vi "autocorrelator-test.vi"() -> ()   [LabVIEW 2011]
uses:
  <vilib>/Waveform/WDTOps.llb/WDT Get XY Value DBL.vi
  <vilib>/Utility/file.llb/Write To Spreadsheet File (DBL).vi
panel:
  in  "file path (dialog if empty)":path
  in  "stop":bool
  out "XY Graph 2":cluster{sgl[], dbl[]}(graph)={[7.5546875, 7.5564947, 7.5579815, 7.559002, 7.5601096, 7.5602555, 7.5602264, 7.559235, 7.5582147, 7.5566406, 7.5546875, 7.552297, 7.5473995, 7.5458837, 7.542823, 7.5388584, 7.534661, 7.530113, 7.524866, 7.519502, 7.5128264, 7.5075793, 7.500583, 7.4940534, 7.4866195, 7.4764752, 7.4705863, 7.4628615, 7.454874, 7.446333, 7.4387536, 7.425752, 7.422225, 7.4146457, 7.4067745, 7.3987875, 7.390654, 7.3826666, 7.3743877, 7.366255, 7.3585587, 7.350513, 7.34238, 7.334655, 7.324598, 7.3181844, 7.310605, 7.302647, 7.294572, 7.286468, 7.274108, 7.270406, 7.2626514, 7.253411, 7.246385, 7.2385726, 7.229361, 7.2227144, 7.2142606, 7.206565, 7.1987233, 7.18922, 7.1825733, 7.1745567, 7.1656075, 7.158582, 7.150449, 7.142607, 7.1346197, 7.1264286, 7.1174207, 7.1103954, 7.102554, 7.0946245, 7.0863748, 7.078533, 7.070633, 7.061917, 7.0544543, 7.046321, 7.038567, 7.0305214, 7.0214844, 7.014138, 7.0066757, 6.997668, 6.9904966, 6.982684, 6.973414, 6.9660974, 6.958576, 6.9507637, 6.942514, 6.9347014, 6.926656, 6.918464, 6.910681, 6.9021688, 6.8945603, 6.8868356, 6.878615, 6.8707733, 6.861299, 6.85474, 6.8466945, 6.838736, 6.8305736, 6.822761, 6.8135204, 6.8067575, 6.798537, 6.7908115, 6.7826786, 6.774662, 6.7665286, 6.7582207, 6.7506413, 6.7427416, 6.7348123, 6.7264752, 6.7184587, 6.7094216, 6.7025127, 6.694584, 6.685372, 6.678667, 6.6677938, 6.661585, 6.65488, 6.6468635, 6.638759, 6.630597, 6.6173334, 6.614331, 6.605848, 6.598414, 6.590631, 6.58276, 6.574773, 6.5666103, 6.557282, 6.5507812, 6.5426483, 6.534923, 6.5267024, 6.5162373, 6.510086, 6.5027695, 6.494549, 6.485337, 6.478603, 6.4657183, 6.4614916, 6.454466, 6.4466243, 6.438841, 6.430679, 6.4228663, 6.4146166, 6.4059877, 6.398904, 6.3908, 6.3826957, 6.374621, 6.364797, 6.357568, 6.350746, 6.341593, 6.334859, 6.326726, 6.314191, 6.310372, 6.3027344, 6.2948346, 6.286789, 6.2786264, 6.2707267, 6.2627683, 6.2544894, 6.246881, 6.2388935, 6.230673, 6.2226853, 6.213328, 6.206711, 6.1988688, 6.189628, 6.1829524, 6.174761, 6.166832, 6.1586695, 6.150799, 6.142345, 6.1345906, 6.126807, 6.118645, 6.110891, 6.1032825, 6.095616, 6.0896106, 6.083401, 6.0774837, 6.071245, 6.0667562], array[204 elements]}
  out "XY Graph":cluster{sgl[], dbl[]}(graph)={[6.06078, 6.0535216, 6.0500236, 6.045476, 6.043464, 6.041482, 6.0394416, 6.0375757, 6.036381, 6.0350103, 6.034865, 6.034748, 6.034486, 6.0351562, 6.036089, 6.0373716, 6.0391793, 6.041278, 6.043523, 6.046642, 6.0500236, 6.053842, 6.059585, 6.062704, 6.0670185, 6.073169, 6.077921, 6.0840716, 6.090223, 6.097569, 6.1042733, 6.11299, 6.119549, 6.127711, 6.135611, 6.144036, 6.1519938, 6.159573, 6.1677647, 6.175694, 6.1847305, 6.194555, 6.1999183, 6.207964, 6.2158055, 6.223764, 6.2316346, 6.2450733, 6.247843, 6.2556844, 6.264255, 6.2716885, 6.279851, 6.2877216, 6.2958837, 6.304046, 6.3117423, 6.3197293, 6.327775, 6.337162, 6.3461404, 6.3521748, 6.361182, 6.367887, 6.3758745, 6.3849697, 6.3967175, 6.400857, 6.4088445, 6.4162197, 6.423974, 6.432865, 6.4400363, 6.4480233, 6.4571185, 6.463882, 6.4719567, 6.4796233, 6.487844, 6.4978137, 6.5056553, 6.511806, 6.5197935, 6.52781, 6.5358267, 6.548274, 6.5519767, 6.5598764, 6.568884, 6.5757055, 6.583897, 6.5943913, 6.600455, 6.608034, 6.6169834, 6.6240964, 6.631938, 6.6409163, 6.647971, 6.6561627, 6.6638002, 6.671758, 6.6798625, 6.689045, 6.699802, 6.7040286, 6.711695, 6.719887, 6.727816, 6.736707, 6.743645, 6.7518363, 6.7603197, 6.767607, 6.775682, 6.7838736, 6.792007, 6.7997026, 6.807836, 6.815736, 6.8237233, 6.8325267, 6.8398438, 6.8513584, 6.857043, 6.8639517, 6.871706, 6.8812094, 6.887739, 6.89561, 6.9042096, 6.911614, 6.920709, 6.9277053, 6.935809, 6.9447002, 6.952542, 6.960267, 6.9682837, 6.975571, 6.9837337, 6.991721, 7.0029445, 7.0082498, 7.015771, 7.0250115, 7.0316, 7.039704, 7.053492, 7.0564365, 7.0637245, 7.0716243, 7.079874, 7.0878325, 7.0962863, 7.10404, 7.1119986, 7.1208024, 7.1276526, 7.13564, 7.1435986, 7.154559, 7.159952, 7.1677938, 7.1756644, 7.1837397, 7.1916103, 7.205049, 7.2078767, 7.2155433, 7.223589, 7.2315764, 7.2408175, 7.2474346, 7.255626, 7.265071, 7.2714844, 7.279734, 7.2875757, 7.2956505, 7.3059993, 7.3134913, 7.319671, 7.3276877, 7.3355002, 7.3436627, 7.3565183, 7.360745, 7.367945, 7.3757286, 7.383804, 7.391587, 7.399691, 7.4075327, 7.4162197, 7.423741, 7.4315534, 7.4397154, 7.447674, 7.4574685, 7.463911, 7.4716067, 7.479419, 7.4873486, 7.4944906, 7.50516, 7.5080166, 7.5155377, 7.5203185, 7.5253906, 7.530113, 7.534923, 7.5392375, 7.543027, 7.5464377, 7.5495276, 7.552064], array[217 elements]}
  out "Waveform Graph 2":sgl[](graph)=[7.5546875, 7.5564947, 7.5579815, 7.559002, 7.5601096, 7.5602555, 7.5602264, 7.559235, 7.5582147, 7.5566406, 7.5546875, 7.552297, 7.5473995, 7.5458837, 7.542823, 7.5388584, 7.534661, 7.530113, 7.524866, 7.519502, 7.5128264, 7.5075793, 7.500583, 7.4940534, 7.4866195, 7.4764752, 7.4705863, 7.4628615, 7.454874, 7.446333, 7.4387536, 7.425752, 7.422225, 7.4146457, 7.4067745, 7.3987875, 7.390654, 7.3826666, 7.3743877, 7.366255, 7.3585587, 7.350513, 7.34238, 7.334655, 7.324598, 7.3181844, 7.310605, 7.302647, 7.294572, 7.286468, 7.274108, 7.270406, 7.2626514, 7.253411, 7.246385, 7.2385726, 7.229361, 7.2227144, 7.2142606, 7.206565, 7.1987233, 7.18922, 7.1825733, 7.1745567, 7.1656075, 7.158582, 7.150449, 7.142607, 7.1346197, 7.1264286, 7.1174207, 7.1103954, 7.102554, 7.0946245, 7.0863748, 7.078533, 7.070633, 7.061917, 7.0544543, 7.046321, 7.038567, 7.0305214, 7.0214844, 7.014138, 7.0066757, 6.997668, 6.9904966, 6.982684, 6.973414, 6.9660974, 6.958576, 6.9507637, 6.942514, 6.9347014, 6.926656, 6.918464, 6.910681, 6.9021688, 6.8945603, 6.8868356, 6.878615, 6.8707733, 6.861299, 6.85474, 6.8466945, 6.838736, 6.8305736, 6.822761, 6.8135204, 6.8067575, 6.798537, 6.7908115, 6.7826786, 6.774662, 6.7665286, 6.7582207, 6.7506413, 6.7427416, 6.7348123, 6.7264752, 6.7184587, 6.7094216, 6.7025127, 6.694584, 6.685372, 6.678667, 6.6677938, 6.661585, 6.65488, 6.6468635, 6.638759, 6.630597, 6.6173334, 6.614331, 6.605848, 6.598414, 6.590631, 6.58276, 6.574773, 6.5666103, 6.557282, 6.5507812, 6.5426483, 6.534923, 6.5267024, 6.5162373, 6.510086, 6.5027695, 6.494549, 6.485337, 6.478603, 6.4657183, 6.4614916, 6.454466, 6.4466243, 6.438841, 6.430679, 6.4228663, 6.4146166, 6.4059877, 6.398904, 6.3908, 6.3826957, 6.374621, 6.364797, 6.357568, 6.350746, 6.341593, 6.334859, 6.326726, 6.314191, 6.310372, 6.3027344, 6.2948346, 6.286789, 6.2786264, 6.2707267, 6.2627683, 6.2544894, 6.246881, 6.2388935, 6.230673, 6.2226853, 6.213328, 6.206711, 6.1988688, 6.189628, 6.1829524, 6.174761, 6.166832, 6.1586695, 6.150799, 6.142345, 6.1345906, 6.126807, 6.118645, 6.110891, 6.1032825, 6.095616, 6.0896106, 6.083401, 6.0774837, 6.071245, 6.0667562]
  out "Waveform Graph":sgl[](graph)=[6.06078, 6.0535216, 6.0500236, 6.045476, 6.043464, 6.041482, 6.0394416, 6.0375757, 6.036381, 6.0350103, 6.034865, 6.034748, 6.034486, 6.0351562, 6.036089, 6.0373716, 6.0391793, 6.041278, 6.043523, 6.046642, 6.0500236, 6.053842, 6.059585, 6.062704, 6.0670185, 6.073169, 6.077921, 6.0840716, 6.090223, 6.097569, 6.1042733, 6.11299, 6.119549, 6.127711, 6.135611, 6.144036, 6.1519938, 6.159573, 6.1677647, 6.175694, 6.1847305, 6.194555, 6.1999183, 6.207964, 6.2158055, 6.223764, 6.2316346, 6.2450733, 6.247843, 6.2556844, 6.264255, 6.2716885, 6.279851, 6.2877216, 6.2958837, 6.304046, 6.3117423, 6.3197293, 6.327775, 6.337162, 6.3461404, 6.3521748, 6.361182, 6.367887, 6.3758745, 6.3849697, 6.3967175, 6.400857, 6.4088445, 6.4162197, 6.423974, 6.432865, 6.4400363, 6.4480233, 6.4571185, 6.463882, 6.4719567, 6.4796233, 6.487844, 6.4978137, 6.5056553, 6.511806, 6.5197935, 6.52781, 6.5358267, 6.548274, 6.5519767, 6.5598764, 6.568884, 6.5757055, 6.583897, 6.5943913, 6.600455, 6.608034, 6.6169834, 6.6240964, 6.631938, 6.6409163, 6.647971, 6.6561627, 6.6638002, 6.671758, 6.6798625, 6.689045, 6.699802, 6.7040286, 6.711695, 6.719887, 6.727816, 6.736707, 6.743645, 6.7518363, 6.7603197, 6.767607, 6.775682, 6.7838736, 6.792007, 6.7997026, 6.807836, 6.815736, 6.8237233, 6.8325267, 6.8398438, 6.8513584, 6.857043, 6.8639517, 6.871706, 6.8812094, 6.887739, 6.89561, 6.9042096, 6.911614, 6.920709, 6.9277053, 6.935809, 6.9447002, 6.952542, 6.960267, 6.9682837, 6.975571, 6.9837337, 6.991721, 7.0029445, 7.0082498, 7.015771, 7.0250115, 7.0316, 7.039704, 7.053492, 7.0564365, 7.0637245, 7.0716243, 7.079874, 7.0878325, 7.0962863, 7.10404, 7.1119986, 7.1208024, 7.1276526, 7.13564, 7.1435986, 7.154559, 7.159952, 7.1677938, 7.1756644, 7.1837397, 7.1916103, 7.205049, 7.2078767, 7.2155433, 7.223589, 7.2315764, 7.2408175, 7.2474346, 7.255626, 7.265071, 7.2714844, 7.279734, 7.2875757, 7.2956505, 7.3059993, 7.3134913, 7.319671, 7.3276877, 7.3355002, 7.3436627, 7.3565183, 7.360745, 7.367945, 7.3757286, 7.383804, 7.391587, 7.399691, 7.4075327, 7.4162197, 7.423741, 7.4315534, 7.4397154, 7.447674, 7.4574685, 7.463911, 7.4716067, 7.479419, 7.4873486, 7.4944906, 7.50516, 7.5080166, 7.5155377, 7.5203185, 7.5253906, 7.530113, 7.534923, 7.5392375, 7.543027, 7.5464377, 7.5495276, 7.552064]
  in  "Scan Range (mm)":sgl=1.5
  in  "Scan Center (mm)":sgl=6.81
  in  "HWSerialNum":i32=83837638
  in  "MG17Motor":refnum<k7>(container)
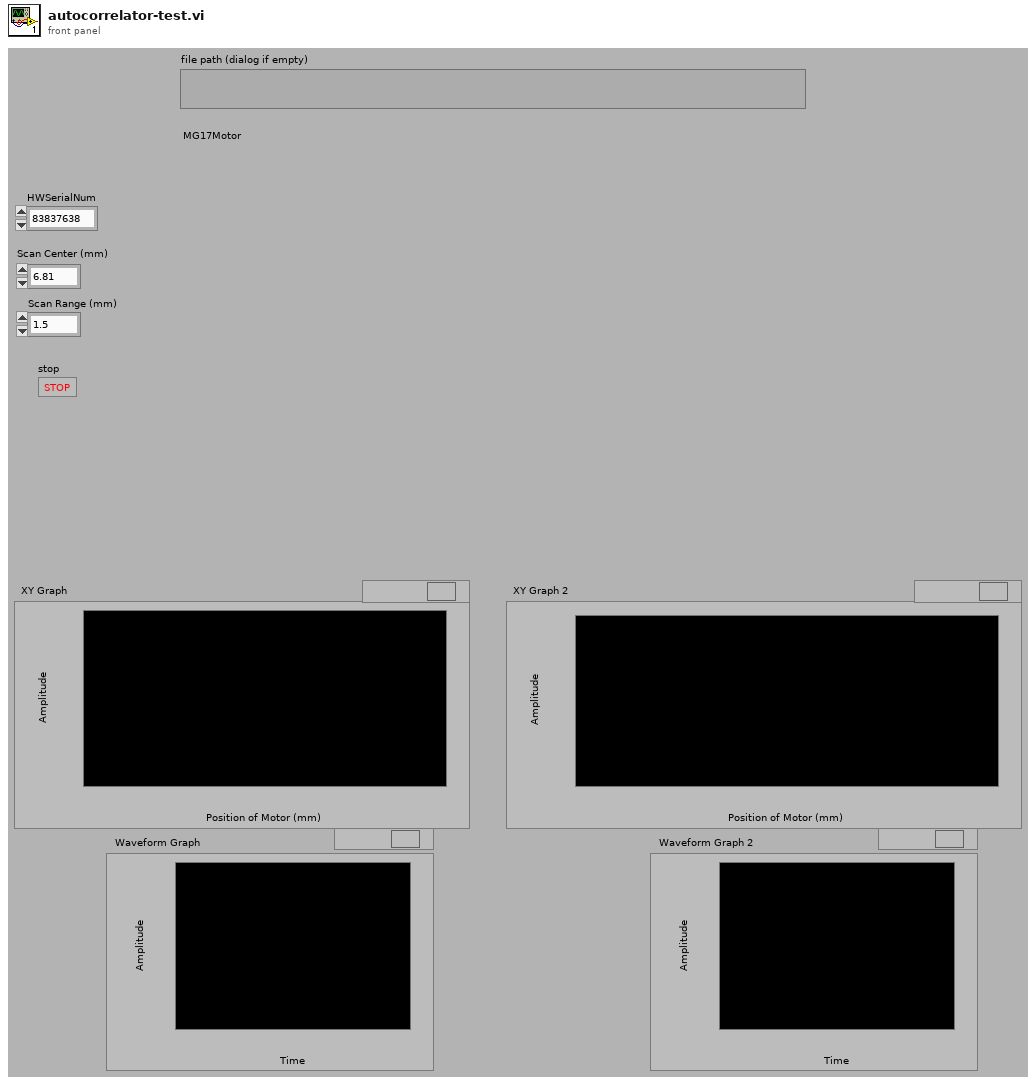
[diagram p1: front panel]
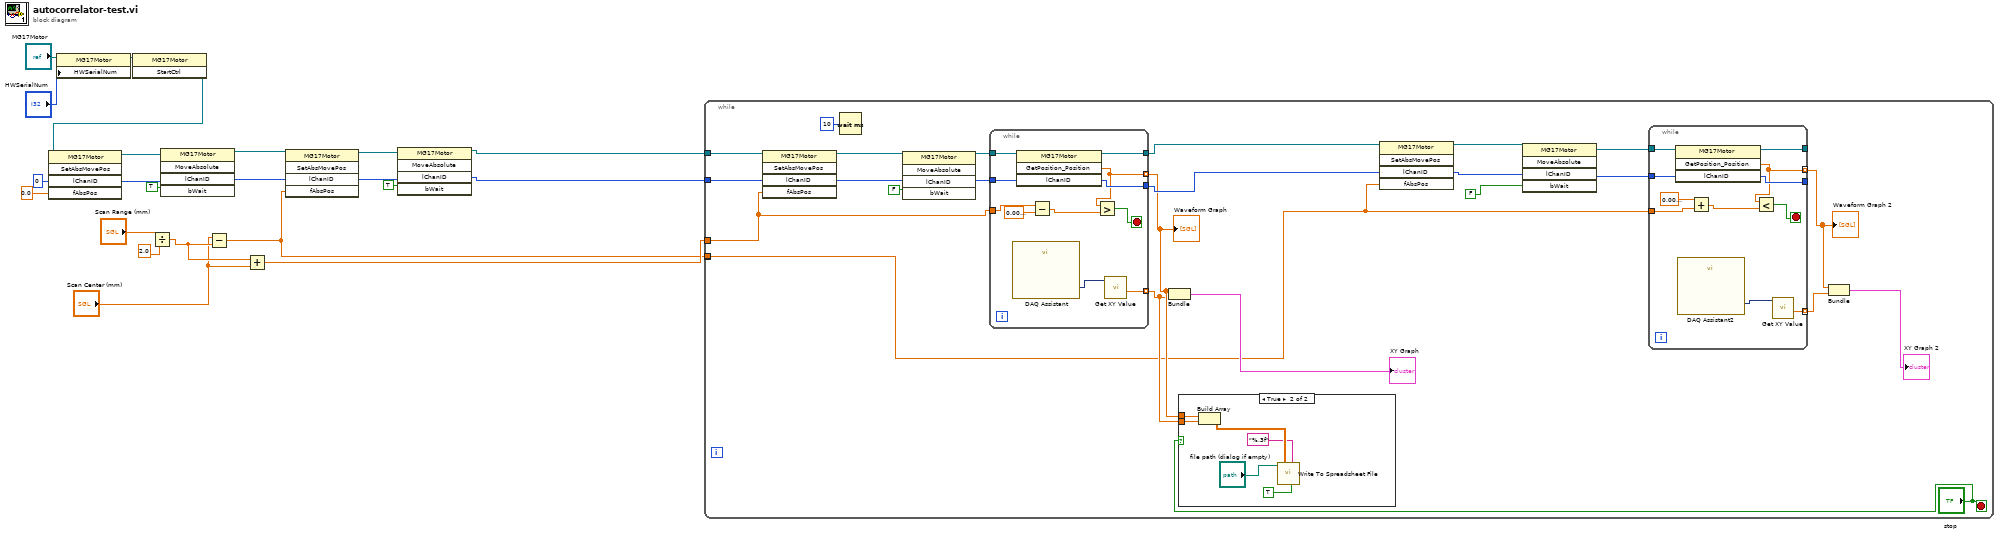
[diagram p0: block diagram]
diagram:
  n1 = property class="MG17Motor"(reference="MG17Motor", "HWSerialNum"="HWSerialNum") -> (reference out=w20:refnum<k7>)  [unwired: 1 in, 1 out]
  n2 = invoke class="MG17Motor" method="StartCtrl"(reference=w20) -> (reference out=w14:refnum<k7>)  [unwired: 2 in, 2 out]
  n3 = invoke class="MG17Motor" method="SetAbsMovePos"(reference=w14, "lChanID"=0, "fAbsPos"=sgl 0.0) -> (reference out=w19:refnum<k7>, "lChanID"=w18:i32)  [unwired: 2 in, 3 out]
  n4 = Divide(x="Scan Range (mm)", y=sgl 2.0) -> (x/y=w4:sgl)
  n5 = invoke class="MG17Motor" method="MoveAbsolute"(reference=w19, "lChanID"=w18, "bWait"=TRUE) -> (reference out=w10:refnum<k7>, "lChanID"=w9:i32)  [unwired: 2 in, 3 out]
  n6 = Subtract(x="Scan Center (mm)", y=w4) -> (x-y=w1:sgl)
  n7 = Add(x=w4, y="Scan Center (mm)") -> (x+y=w2:sgl)
  n8 = invoke class="MG17Motor" method="SetAbsMovePos"(reference=w10, "lChanID"=w9, "fAbsPos"=w1) -> (reference out=w13:refnum<k7>, "lChanID"=w12:i32)  [unwired: 2 in, 3 out]
  n9 = invoke class="MG17Motor" method="MoveAbsolute"(reference=w13, "lChanID"=w12, "bWait"=TRUE) -> (reference out=w8:refnum<k7>, "lChanID"=w7:i32)  [unwired: 2 in, 3 out]
  n10 = while {
    tunnel: w8 -> [w43]
    tunnel: w7 -> [w42]
    tunnel: w2 -> [w31]
    tunnel: [w24] -> _
    tunnel: w1 -> [w24]
    stop <- "stop" stop-if-true
    n11 = invoke class="MG17Motor" method="SetAbsMovePos"(reference=w43, "lChanID"=w42, "fAbsPos"=w31) -> (reference out=w45:refnum<k7>, "lChanID"=w44:i32)  [unwired: 2 in, 3 out]
    n12 = Wait (ms)(milliseconds to wait=u32 10) -> ()  [unwired: 1 out]
    n13 = invoke class="MG17Motor" method="MoveAbsolute"(reference=w45, "lChanID"=w44, "bWait"=FALSE) -> (reference out=w40:refnum<k7>, "lChanID"=w41:i32)  [unwired: 2 in, 3 out]
    n14 = while {
      tunnel: w41 -> [w74]
      tunnel: w40 -> [w73]
      tunnel: [w70] -> w26 mode=indexing
      tunnel: [w72] -> w35
      tunnel: [w71] -> w34
      tunnel: w31 -> [w69]
      tunnel: [w64] -> w25 mode=indexing
      stop <- w66 stop-if-true
      n15 = call "DAQ Assistant"() -> ("data"=w65:dynamicdata)  [unwired: 17 in, 2 out]
      n16 = invoke class="MG17Motor" method="GetPosition_Position"(reference=w73, "lChanID"=w74) -> (reference out=w72:refnum<k7>, "GetPosition_Position"=w70:sgl, "lChanID"=w71:i32)  [unwired: 2 in, 1 out]
      n17 = Subtract(x=w69, y=sgl 0.01) -> (x-y=w67:sgl)
      n18 = Greater?(x=w70, y=w67) -> (0:w66:bool)
      n19 = call-poly <vilib>:"Get XY Value.vi"("waveform in"=w65) -> ("Y value"=w64:dbl)  [unwired: 6 in, 4 out]
    }
    "Waveform Graph" <- w26
    n20 = Bundle(w26, w25) -> (→"XY Graph":cluster{sgl[], dbl[]})  [unwired: 1 in]
    n21 = case shown="True" "stop" {
      tunnel: w26 -> [_ w52]
      tunnel: w25 -> [_ w51]
      frame False {
      }
      frame True {
        n22 = Build Array(w52, w51) -> (w50:dbl[][])
        n23 = call-poly <vilib>:"Write To Spreadsheet File.vi"("transpose? (no:F)"=TRUE, "format (%.3f)"="%.3f", "2D data"=w50, "file path (dialog if empty)"="file path (dialog if empty)") -> ()  [unwired: 4 in, 1 out]
      }
    }
    n24 = invoke class="MG17Motor" method="SetAbsMovePos"(reference=w35, "lChanID"=w34, "fAbsPos"=w24) -> (reference out=w38:refnum<k7>, "lChanID"=w36:i32)  [unwired: 2 in, 3 out]
    n25 = invoke class="MG17Motor" method="MoveAbsolute"(reference=w38, "lChanID"=w36, "bWait"=FALSE) -> (reference out=w33:refnum<k7>, "lChanID"=w32:i32)  [unwired: 2 in, 3 out]
    n26 = while {
      tunnel: w32 -> [w63]
      tunnel: w33 -> [w62]
      tunnel: [w59] -> w29 mode=indexing
      tunnel: [w61] -> _
      tunnel: [w60] -> _
      tunnel: w24 -> [w55]
      tunnel: [w53] -> w28 mode=indexing
      stop <- w57 stop-if-true
      n27 = invoke class="MG17Motor" method="GetPosition_Position"(reference=w62, "lChanID"=w63) -> (reference out=w61:refnum<k7>, "GetPosition_Position"=w59:sgl, "lChanID"=w60:i32)  [unwired: 2 in, 1 out]
      n28 = call "DAQ Assistant2"() -> ("data"=w54:dynamicdata)  [unwired: 17 in, 2 out]
      n29 = Add(x=sgl 0.01 ("y"), y=w55) -> (x+y=w58:sgl)
      n30 = Less?(x=w59, y=w58) -> (x < y?=w57:bool)
      n31 = call-poly <vilib>:"Get XY Value.vi"("waveform in"=w54) -> ("Y value"=w53:dbl)  [unwired: 6 in, 4 out]
    }
    "Waveform Graph 2" <- w29
    n32 = Bundle(w29, w28) -> (→"XY Graph 2":cluster{sgl[], dbl[]})  [unwired: 1 in]
  }
